vi "Receive Topic Message.vi"(7 "Websocket Topic Actor in":refnum<class "Websocket Topic Actor.lvclass">, 8 "error in (no error)":errorcluster, 10 "Message in":refnum<class "Message Interface.lvclass">) -> (0 "error out":errorcluster, 3 "Stop?":bool, 5 "Websocket Topic Actor out":refnum<class "Websocket Topic Actor.lvclass">)   [LabVIEW 2016, in "Stream Mediator.lvlib" / "Websocket Topic Actor.lvclass"]
doc: "--\nCopyright © 2017 Composed SystemsI All rights reserved.\n\nAuthor: Jon McBee <jon.mcbee@composed.io>\n\nThis library is provided \"AS IS\" ,WITHOUT WARRANTIES OR\nCONDITIONS OF ANY KIND, either express or implied.\n\nComposed Systems -- composed.io\n\nStream 0.0.1.1\nJon McBee - Composed Systems\nCopyright (c) 2017, Composed Systems"
uses:
  <userlib>/Composed Systems/Stream/Mediator/Classes/Websocket Topic Actor/Websocket Topic Actor.lvclass
  <userlib>/Composed Systems/Stream/Mediator/Classes/Message Interface/Message Interface.lvclass
  <userlib>/Composed Systems/Stream/Mediator/Classes/Topic Actor/Topic Actor.lvclass
  <userlib>/Composed Systems/Stream/Mediator/Classes/Topic Actor Command Interface/Topic Actor Command Interface.lvclass
  <userlib>/Composed Systems/Stream/Mediator/Classes/Message Transport Queue/Message Transport Queue.lvclass
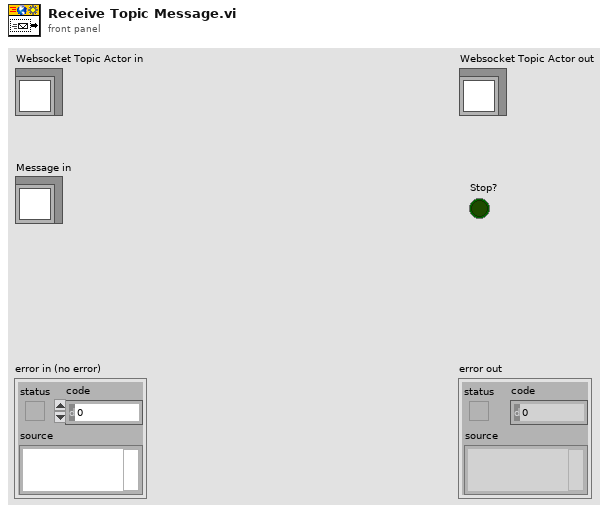
[diagram p1: front panel]
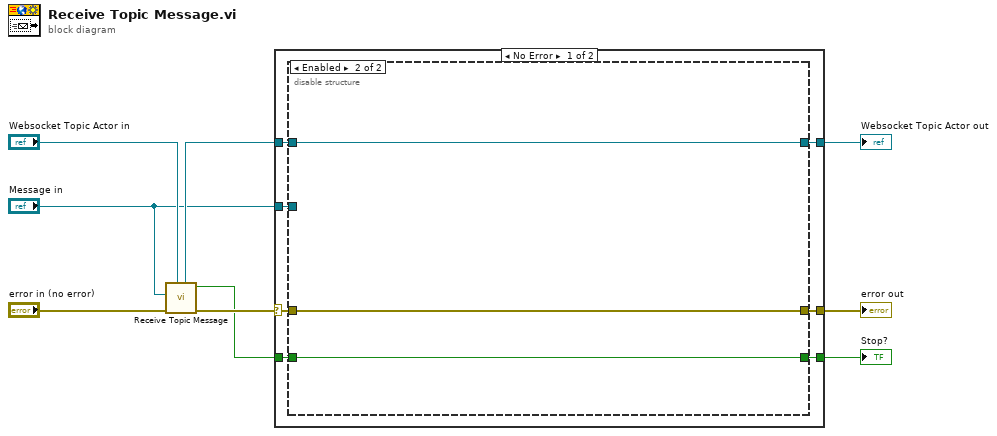
[diagram p0: block diagram]
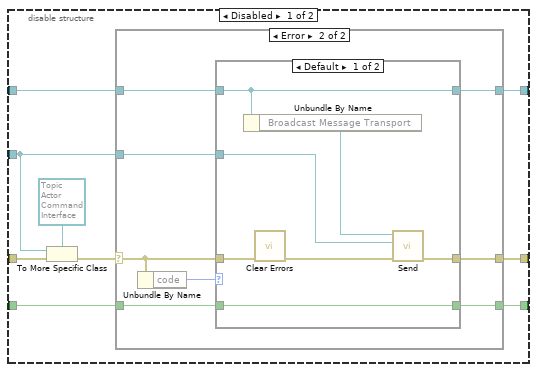
[diagram p2: hidden frame]
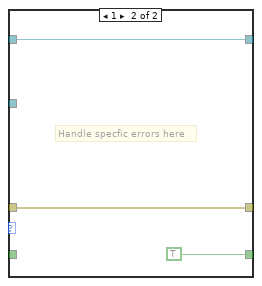
[diagram p4: hidden frame]
diagram:
  n1 = call-parent "Receive Topic Message.vi"("Topic Actor in"="Websocket Topic Actor in", "error in (no error)"="error in (no error)", "Message in"="Message in") -> ("error out"=w7:errorcluster, "Stop?"=w2:bool, "Topic Actor out"=w5:refnum<class "Websocket Topic Actor.lvclass">)  [unwired: 6 in]
  n2 = case shown="No Error" w7 {
    selector: w7 -> [w16 w51]
    tunnel: [w13 w51] -> w6
    tunnel: [w14 w52] -> w4
    tunnel: w5 -> [w15 w52]
    tunnel: "Message in" -> [w10 _]
    tunnel: w2 -> [w12 w50]
    tunnel: [w11 w50] -> w1
    frame No Error {
      n3 = disable-structure shown="Enabled" {
        disable-tunnel: w16 -> [w24 w48]
        disable-tunnel: w15 -> [w22 w49]
        disable-tunnel: [w21 w49] -> w14
        disable-tunnel: [w20 w48] -> w13
        disable-tunnel: w12 -> [w19 w47]
        disable-tunnel: [w18 w47] -> w11
        disable-tunnel: w10 -> [w17 _]
        frame Disabled {
          n4 = To More Specific Class(target class=refnum<class "Topic Actor Command Interface.lvclass"> refnum ("Topic Actor Command Interface.lvclass"), reference=w17, error in=w24) -> (error out=w23:errorcluster)  [unwired: 1 out]
          n5 = case shown="Error" w23 {
            selector: w23 -> [w26 w32]
            tunnel: [w28 w34] -> w21
            tunnel: w22 -> [w28 w35]
            tunnel: [w26 w33] -> w20
            tunnel: w19 -> [w27 w31]
            tunnel: [w27 w30] -> w18
            tunnel: w17 -> [_ w29]
            frame No Error {
            }
            frame Error {
              n6 = Unbundle By Name(w32) -> ("code"=w36:i32)
              n7 = case shown="Default" w36 {
                tunnel: w35 -> [w41 w46]
                tunnel: [w41 w46] -> w34
                tunnel: [w38 w45] -> w33
                tunnel: w32 -> [w42 w45]
                tunnel: w31 -> [w43 _]
                tunnel: [w43 TRUE ("Stop?")] -> w30
                tunnel: w29 -> [w37 _]
                frame Default {
                  n8 = Unbundle By Name(w41) -> ("Broadcast Message Transport"=w40:refnum<class "Message Transport Queue.lvclass">)
                  n9 = call <vilib>:"Clear Errors.vi"("error in (no error)"=w42) -> ("error out"=w39:errorcluster)  [unwired: 5 in, 1 out]
                  n10 = call-dynamic "Send.vi"("error in (no error)"=w39, "Message"=w37, "Message Transport Queue in"=w40) -> ("error out"=w38:errorcluster)  [unwired: 6 in, 2 out]
                }
                frame 1 {
                  # "Handle specfic errors here"
                }
              }
            }
          }
        }
        frame Enabled {
        }
      }
    }
    frame Error {
    }
  }
  "error out" <- w6
  "Websocket Topic Actor out" <- w4
  "Stop?" <- w1
